vi "PQdsplen.vi"(8 "error in (no error)":errorcluster, 10 "encoding":i32, 11 "s":string) -> (0 "error out":errorcluster, 3 "return type":i32)   [LabVIEW 2019, in "libpqlv64.lvlib"]
uses:
  libpqlv64.lvlib
  libpq.dll
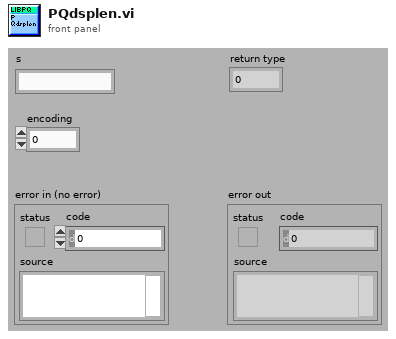
[diagram p1: front panel]
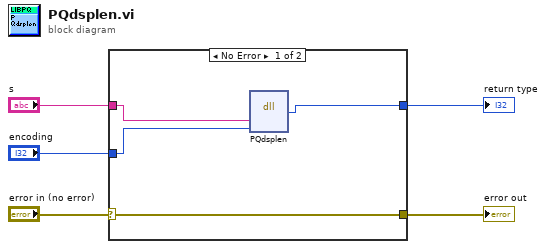
[diagram p0: block diagram]
diagram:
  n1 = case shown="No Error" "error in (no error)" {
    selector: "error in (no error)" -> [w9 w10]
    tunnel: [w9 w10] -> w4
    tunnel: [w8 _] -> w3
    tunnel: "s" -> [w7 _]
    tunnel: "encoding" -> [w6 _]
    frame No Error {
      n2 = dll-call lib="libpq.*" fn="PQdsplen"("s"=w7, "encoding"=w6) -> (w8:i32)  [unwired: 5 in, 2 out]
    }
    frame Error {
    }
  }
  "return type" <- w3
  "error out" <- w4
